vi "Config Main Error&Alarm.vi"(8 "error in (no error)":errorcluster, 11 "Sequence":T1) -> (0 "error out":errorcluster, 3 "Sequence out":T1)   [LabVIEW 2014, in "SeqLoop.lvlib"]
uses:
  TypeDefs/Sequence.ctl
  TypeDefs/STEP.ctl
  TypeDefs/LogicParsedExpression.ctl
  Mimico Display/TypeDefs/Mimic Data.ctl
  Mimico Display/TypeDefs/BG Image.ctl
  Mimico Display/TypeDefs/mObject.ctl
  <vilib>/regexp/Match Regular Expression.xnode
  SeqLoop.lvlib
  Mimico Display/Mimico Display.lvlib
panel:
  in  "Mensaje de Error":string
  in  "Alarm Msj 4":string
  in  "Alarm Msj 3":string
  in  "Alarm Msj 2":string
  in  "Alarm Msj 1":string
  in  "Alarm 4":string
  in  "Alarm 3":string
  in  "Alarm 2":string
  in  "Alarm 1":string
  in  "Condición de Error":string
  in  "Stop Med":bool
  in  "Add Med":bool
  # "Alarma"
  # "Mensaje de Alarma"
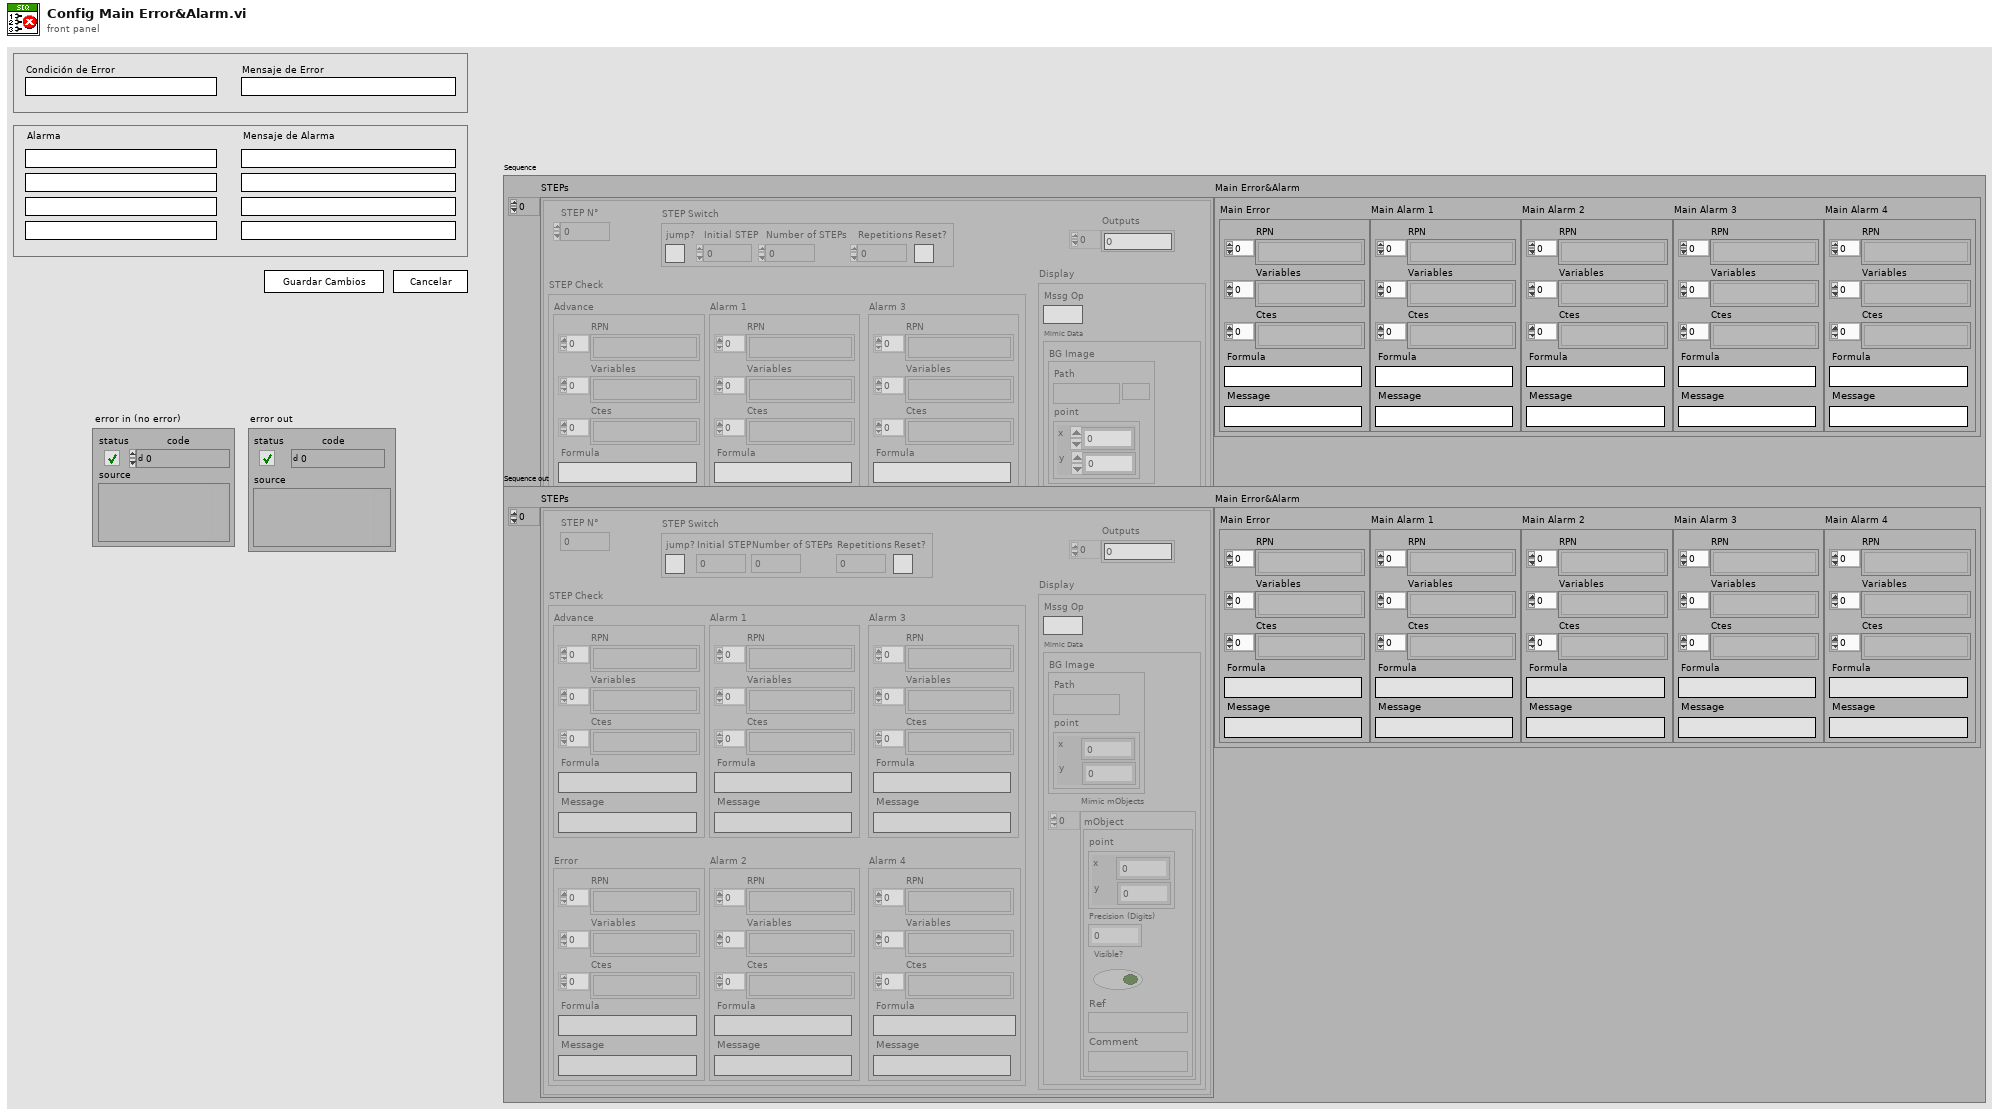
[diagram p1: front panel]
types:
  T1 = typedef "SeqLoop.lvlib/Sequence.ctl" = cluster{"STEPs":T2[], "Main Error&Alarm":cluster{"Main Error":T3, "Main Alarm 1":T3, "Main Alarm 2":T3, "Main Alarm 3":T3, "Main Alarm 4":T3}}
  T2 = typedef "SeqLoop.lvlib/STEP.ctl" = cluster{"STEP N°":u32, "STEP Switch":cluster{"jump?":bool, "Initial STEP":u32, "Number of STEPs":u32, "Repetitions":u32, "Reset?":bool}, "Outputs":i32[], "STEP Check":cluster{"Advance":T3, "Error ":T3, "Alarm 1":T3, "Alarm 2":T3, "Alarm 3":T3, "Alarm 4":T3}, "Display":cluster{"Mssg Op":string, "Mimic Data":T4}}
  T3 = typedef "SeqLoop.lvlib/LogicParsedExpression.ctl" = cluster{"RPN ":string[], "Variables":string[], "Ctes":string[], "Formula":string, "Message":string}
  T4 = typedef "SeqLoop.lvlib/Mimico Display.lvlib/Mimic Data.ctl" = cluster{"BG Image":T5, "Mimic mObjects":T6[]}
  T5 = typedef "SeqLoop.lvlib/Mimico Display.lvlib/BG Image.ctl" = cluster{"Path":path, "point":cluster{"x":i16, "y":i16}}
  T6 = typedef "SeqLoop.lvlib/Mimico Display.lvlib/mObject.ctl" = cluster{"point":cluster{"x":i16, "y":i16}, "Precision (Digits)":i32, "Visible?":bool, "Ref":string, "Comment":string}
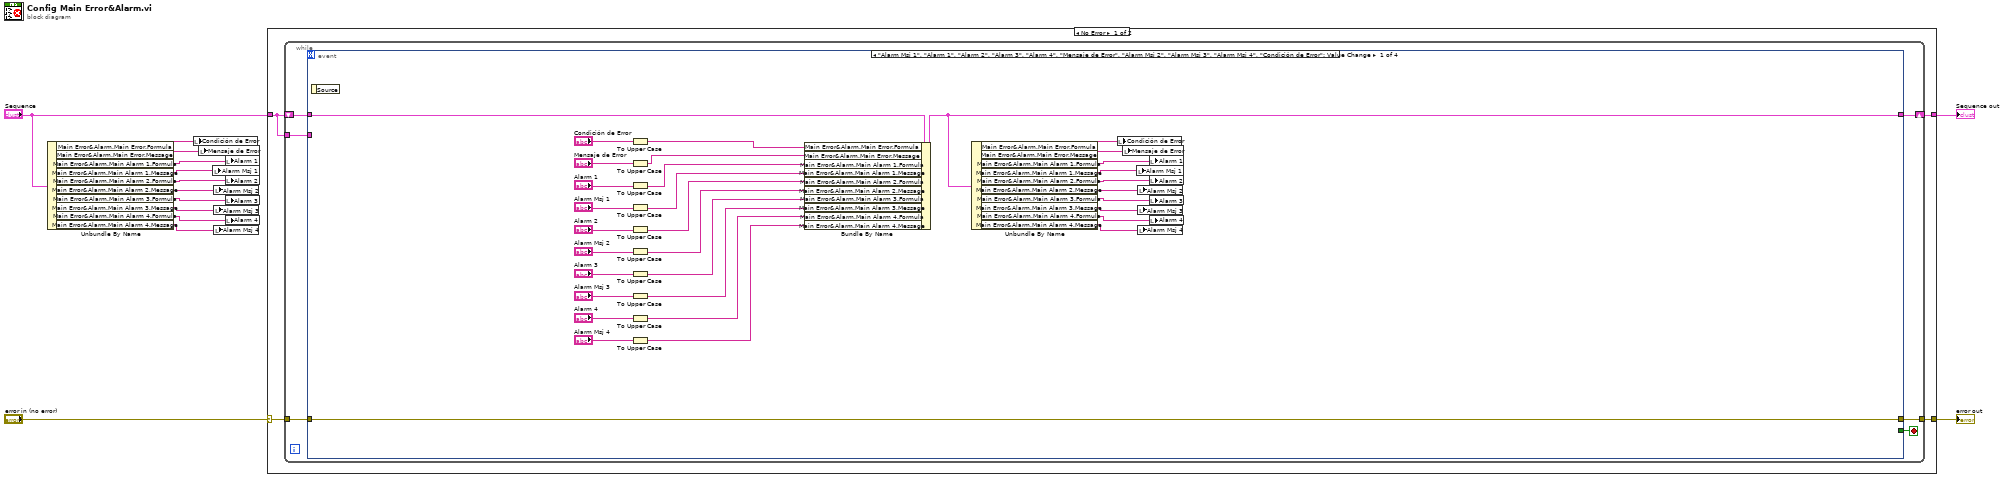
[diagram p0: block diagram]
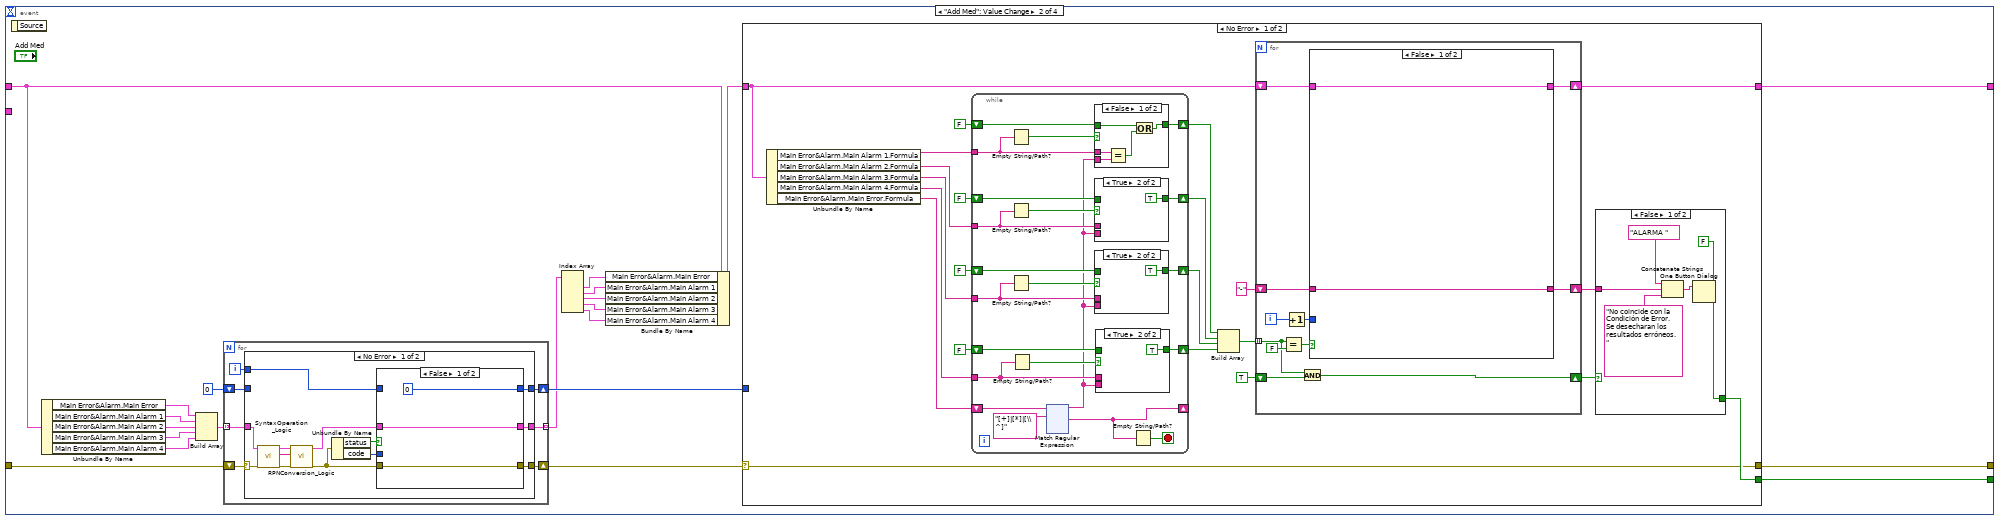
[diagram p2: hidden frame]
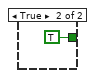
[diagram p3: hidden frame]
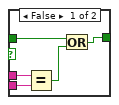
[diagram p4: hidden frame]
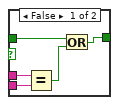
[diagram p5: hidden frame]
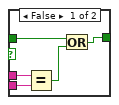
[diagram p6: hidden frame]
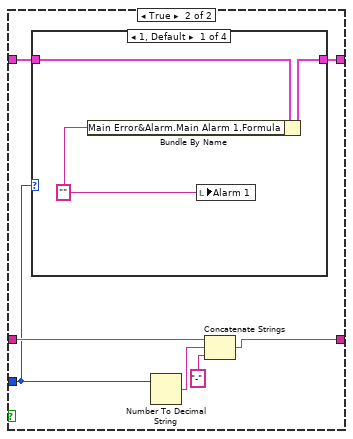
[diagram p7: hidden frame]
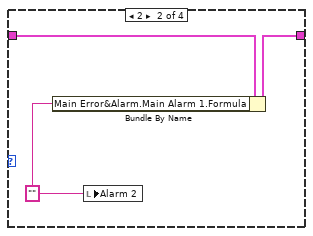
[diagram p8: hidden frame]
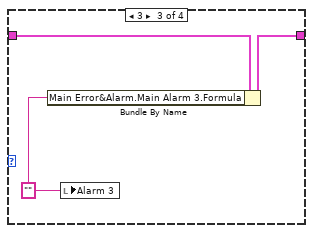
[diagram p9: hidden frame]
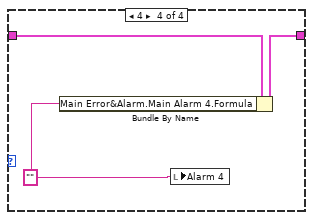
[diagram p10: hidden frame]
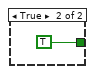
[diagram p11: hidden frame]
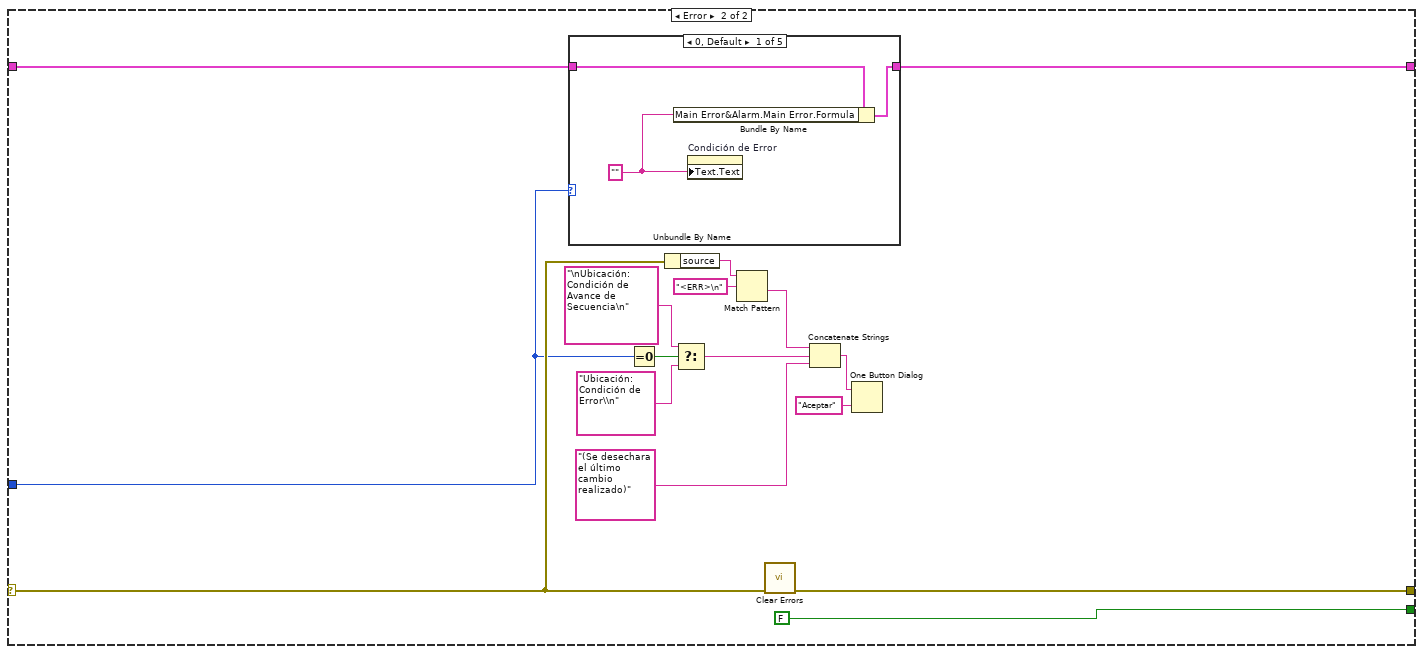
[diagram p12: hidden frame]
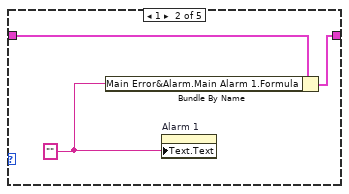
[diagram p13: hidden frame]
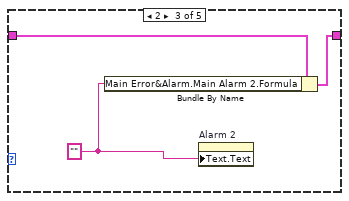
[diagram p14: hidden frame]
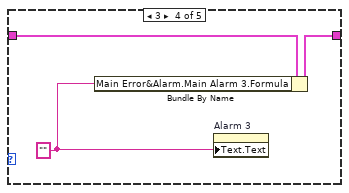
[diagram p15: hidden frame]
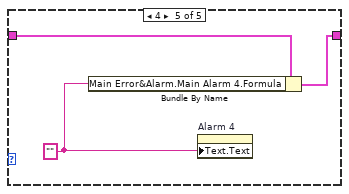
[diagram p16: hidden frame]
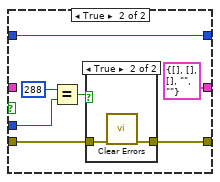
[diagram p17: hidden frame]
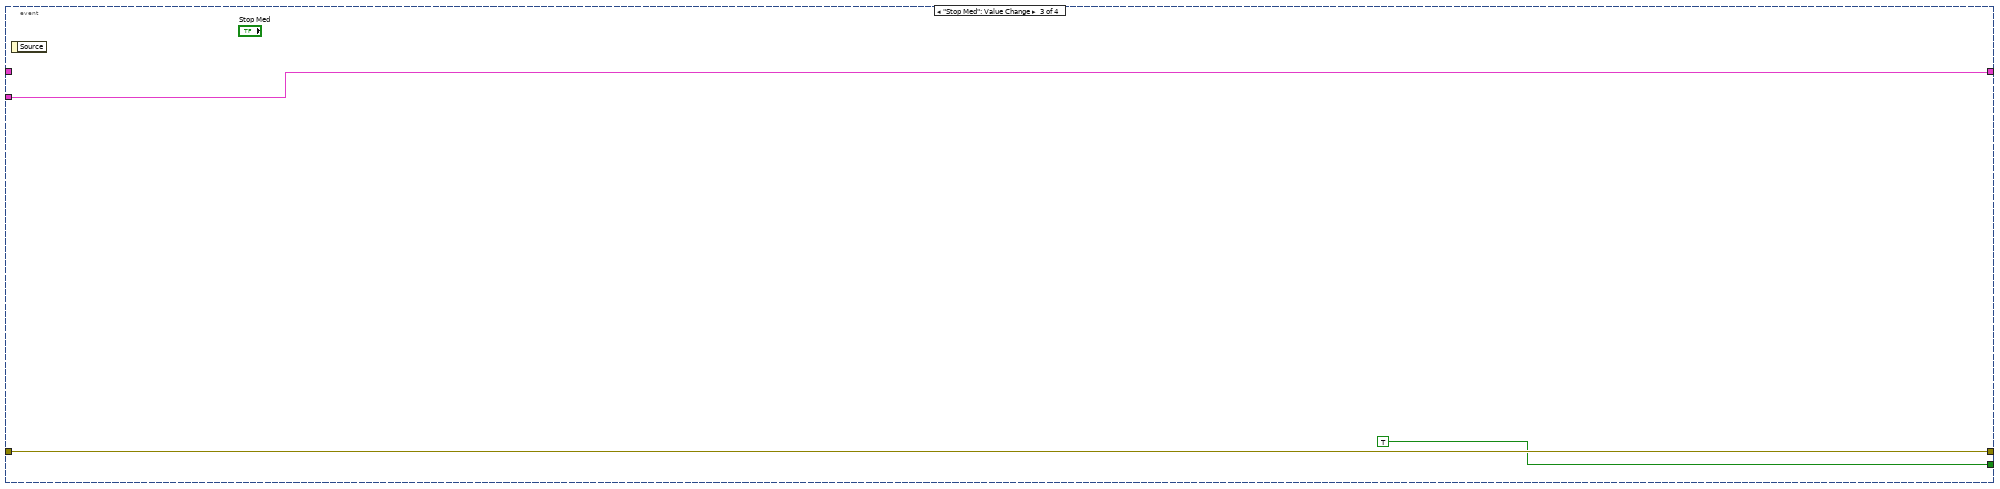
[diagram p20: hidden frame]
diagram:
  n1 = Unbundle By Name("Sequence") -> ("Main Error&Alarm.Main Error.Formula"=w11:string, "Main Error&Alarm.Main Error.Message"=w10:string, "Main Error&Alarm.Main Alarm 1.Formula"=w6:string, "Main Error&Alarm.Main Alarm 1.Message"=w5:string, "Main Error&Alarm.Main Alarm 2.Formula"=w4:string, "Main Error&Alarm.Main Alarm 2.Message"=w3:string, "Main Error&Alarm.Main Alarm 3.Formula"=w2:string, "Main Error&Alarm.Main Alarm 3.Message"=w7:string, "Main Error&Alarm.Main Alarm 4.Formula"=w8:string, "Main Error&Alarm.Main Alarm 4.Message"=w9:string)
  n2 = local write "Condición de Error"(w11) -> ()
  n3 = local write "Mensaje de Error"(w10) -> ()
  n4 = local write "Alarm Msj 1"(w5) -> ()
  n5 = local write "Alarm Msj 2"(w3) -> ()
  n6 = local write "Alarm Msj 3"(w7) -> ()
  n7 = local write "Alarm Msj 4"(w9) -> ()
  n8 = local write "Alarm 1"(w6) -> ()
  n9 = local write "Alarm 2"(w4) -> ()
  n10 = local write "Alarm 3"(w2) -> ()
  n11 = local write "Alarm 4"(w8) -> ()
  n12 = case shown="No Error" "error in (no error)" {
    selector: "error in (no error)" -> [w18 w373]
    tunnel: [w17 w373] -> w13
    tunnel: "Sequence" -> [w15 w372]
    tunnel: [w16 w372] -> w12
    frame No Error {
      n13 = while {
        tunnel: w18 -> [w24]
        tunnel: [w23] -> w17
        shift-right: [w19] -> w16
        shift-left: w15 -> [w21]
        tunnel: w15 -> [w20]
        stop <- w22 stop-if-true
        n14 = event shown="[0] \"Alarm Msj 1\", \"Alarm 1\", \"Alarm 2\", \"Alarm 3\", \"Alarm 4\", \"Mensaje de Error\", \"Alarm Msj 2\", \"Alarm Msj 3\", \"Alarm Msj 4\", \"Condición de Error\": Value Change" {
          selector: _ -> [_ _ _ _]
          dyn-events: _ -> [_ _ _ _]
          timeout: _ -> [_ _ _ _]
          tunnel: w24 -> [w57 w69 w366 w369]
          tunnel: [w57 w66 w366 w369] -> w23
          tunnel: [_ w68 TRUE ("Discard?") TRUE ("Discard?")] -> w22
          tunnel: w21 -> [w56 w65 _ _]
          tunnel: w20 -> [_ _ w367 w368]
          tunnel: [w45 w67 w367 w368] -> w19
          event "Alarm Msj 1", "Alarm 1", "Alarm 2", "Alarm 3", "Alarm 4", "Mensaje de Error", "Alarm Msj 2", "Alarm Msj 3", "Alarm Msj 4", "Condición de Error": Value Change {
            n15 = event-data() -> ()  [unwired: 1 in, 1 out]
            n16 = To Upper Case(1:"Condición de Error") -> (0:w25:string)
            n17 = To Upper Case(1:"Mensaje de Error") -> (0:w27:string)
            n18 = To Upper Case(1:"Alarm 1") -> (0:w29:string)
            n19 = To Upper Case(1:"Alarm Msj 1") -> (0:w31:string)
            n20 = To Upper Case(1:"Alarm 2") -> (0:w33:string)
            n21 = To Upper Case(1:"Alarm Msj 2") -> (0:w35:string)
            n22 = To Upper Case(1:"Alarm 3") -> (0:w37:string)
            n23 = To Upper Case(1:"Alarm Msj 3") -> (0:w39:string)
            n24 = To Upper Case(1:"Alarm 4") -> (0:w41:string)
            n25 = To Upper Case(1:"Alarm Msj 4") -> (0:w43:string)
            n26 = Bundle By Name(cluster=w56, "Main Error&Alarm.Main Error.Formula"=w25, "Main Error&Alarm.Main Error.Message"=w27, "Main Error&Alarm.Main Alarm 1.Formula"=w29, "Main Error&Alarm.Main Alarm 1.Message"=w31, "Main Error&Alarm.Main Alarm 2.Formula"=w33, "Main Error&Alarm.Main Alarm 2.Message"=w35, "Main Error&Alarm.Main Alarm 3.Formula"=w37, "Main Error&Alarm.Main Alarm 3.Message"=w39, "Main Error&Alarm.Main Alarm 4.Formula"=w41, "Main Error&Alarm.Main Alarm 4.Message"=w43) -> (w45:T1)
            n27 = Unbundle By Name(w45) -> ("Main Error&Alarm.Main Error.Formula"=w46:string, "Main Error&Alarm.Main Error.Message"=w47:string, "Main Error&Alarm.Main Alarm 1.Formula"=w51:string, "Main Error&Alarm.Main Alarm 1.Message"=w52:string, "Main Error&Alarm.Main Alarm 2.Formula"=w53:string, "Main Error&Alarm.Main Alarm 2.Message"=w54:string, "Main Error&Alarm.Main Alarm 3.Formula"=w55:string, "Main Error&Alarm.Main Alarm 3.Message"=w50:string, "Main Error&Alarm.Main Alarm 4.Formula"=w49:string, "Main Error&Alarm.Main Alarm 4.Message"=w48:string)
            n28 = local write "Condición de Error"(w46) -> ()
            n29 = local write "Mensaje de Error"(w47) -> ()
            n30 = local write "Alarm Msj 1"(w52) -> ()
            n31 = local write "Alarm Msj 2"(w54) -> ()
            n32 = local write "Alarm Msj 3"(w50) -> ()
            n33 = local write "Alarm Msj 4"(w48) -> ()
            n34 = local write "Alarm 1"(w51) -> ()
            n35 = local write "Alarm 2"(w53) -> ()
            n36 = local write "Alarm 3"(w55) -> ()
            n37 = local write "Alarm 4"(w49) -> ()
          }
          event "Add Med": Value Change {
            n38 = event-data() -> ()  [unwired: 1 in, 1 out]
            n39 = Unbundle By Name(w65) -> ("Main Error&Alarm.Main Error"=w78:T3, "Main Error&Alarm.Main Alarm 1"=w77:T3, "Main Error&Alarm.Main Alarm 2"=w76:T3, "Main Error&Alarm.Main Alarm 3"=w75:T3, "Main Error&Alarm.Main Alarm 4"=w74:T3)
            n40 = Build Array(w78, w77, w76, w75, w74) -> (w70:T3[])
            n41 = for {
              tunnel: w70 -> [w335] mode=indexing
              shift-right: [w334] -> w73
              shift-left: w69 -> [w332]
              shift-right: [w331] -> w72
              shift-left: 0 -> [w330]
              tunnel: [w329] -> w63 mode=indexing
              i -> [w333]
              n42 = case shown="No Error" w332 {
                selector: w332 -> [w345 w364]
                tunnel: w335 -> [w342 w362]
                tunnel: [w347 w364] -> w334
                tunnel: w333 -> [w346 _]
                tunnel: [w344 w363] -> w331
                tunnel: w330 -> [_ w363]
                tunnel: [w336 w362] -> w329
                frame No Error {
                  n43 = call "SyntaxOperation_Logic.vi"("error in (no error)"=w345, "Logical Parsed Expression"=w342) -> ("error out"=w341:errorcluster, "Token"=w339:string[], "Logical Parsed Expression Out"=w338:T3)  [unwired: 6 in, 1 out]
                  n44 = call "RPNConversion_Logic.vi"("error in"=w341, "Token"=w339, "Logical Parsed Expression"=w338) -> ("error out"=w340:errorcluster, "Logical Parsed Expression Out"=w337:T3)  [unwired: 7 in]
                  n45 = Unbundle By Name(w340) -> ("status"=w348:bool, "code"=w343:i32)
                  n46 = case shown="False" w348 {
                    tunnel: [w351 w353] -> w347
                    tunnel: w340 -> [w351 w354]
                    tunnel: w346 -> [_ w358]
                    tunnel: [0 w358] -> w344
                    tunnel: w343 -> [_ w357]
                    tunnel: w337 -> [w349 _]
                    tunnel: [w349 T3 {"RPN "=[], "Variables"=[], "Ctes"=[], "Formula"="", "Message"=""} ("Logical Parsed Expression Out")] -> w336
                    frame False {
                    }
                    frame True {
                      n47 = Equal?(x=288, y=w357) -> (x = y?=w355:bool)
                      n48 = case shown="True" w355 {
                        tunnel: w354 -> [w359 w361]
                        tunnel: [w359 w360] -> w353
                        frame False {
                        }
                        frame True {
                          n49 = call <vilib>:"Clear Errors.vi"("error in (no error)"=w361) -> ("error out"=w360:errorcluster)  [unwired: 5 in, 1 out]
                        }
                      }
                    }
                  }
                }
                frame Error {
                }
              }
            }
            n50 = Index Array(array=w63) -> (element #1=w62:T3, element #2=w59:T3, element #3=w58:T3, element #4=w60:T3, element #5=w61:T3)  [unwired: 5 in]
            n51 = Bundle By Name(cluster=w65, "Main Error&Alarm.Main Error"=w62, "Main Error&Alarm.Main Alarm 1"=w59, "Main Error&Alarm.Main Alarm 2"=w58, "Main Error&Alarm.Main Alarm 3"=w60, "Main Error&Alarm.Main Alarm 4"=w61) -> (w64:T1)
            n52 = case shown="No Error" w73 {
              selector: w73 -> [w85 w308]
              tunnel: [w96 w304] -> w67
              tunnel: w64 -> [w84 w305]
              tunnel: [w85 w307] -> w66
              tunnel: [w95 FALSE ("Discard?")] -> w68
              tunnel: w72 -> [_ w301]
              frame No Error {
                n53 = Unbundle By Name(w84) -> ("Main Error&Alarm.Main Alarm 1.Formula"=w83:string, "Main Error&Alarm.Main Alarm 2.Formula"=w82:string, "Main Error&Alarm.Main Alarm 3.Formula"=w81:string, "Main Error&Alarm.Main Alarm 4.Formula"=w80:string, "Main Error&Alarm.Main Error.Formula"=w79:string)
                n54 = while {
                  shift-right: [w101] -> _
                  shift-left: w79 -> [w103]
                  tunnel: w80 -> [w120]
                  tunnel: w81 -> [w113]
                  tunnel: w82 -> [w112]
                  tunnel: w83 -> [w111]
                  shift-right: [w119] -> w87
                  shift-left: FALSE -> [w118]
                  shift-right: [w108] -> w88
                  shift-left: FALSE -> [w105]
                  shift-right: [w109] -> w89
                  shift-left: FALSE -> [w106]
                  shift-right: [w110] -> w90
                  shift-left: FALSE -> [w107]
                  stop <- w117 stop-if-true
                  n55 = Empty String/Path?(string/path=w111) -> (empty?=w114:bool)
                  n56 = Empty String/Path?(string/path=w112) -> (empty?=w115:bool)
                  n57 = Empty String/Path?(string/path=w113) -> (empty?=w116:bool)
                  n58 = Empty String/Path?(string/path=w120) -> (empty?=w121:bool)
                  n59 = xnode "Match Regular Expression"("input string"=w103, "regular expression"="[+]|[*]|[\\^]") -> ("before match"=w102:string, "after match"=w101:string)  [unwired: 4 in, 3 out]
                  n60 = case shown="False" w114 {
                    tunnel: w111 -> [w240 _]
                    tunnel: w102 -> [w239 _]
                    tunnel: w107 -> [w238 _]
                    tunnel: [w236 TRUE] -> w110
                    frame False {
                      n61 = Equal?(x=w240, y=w239) -> (x = y?=w237:bool)
                      n62 = Or(x=w238, y=w237) -> (x .or. y?=w236:bool)
                    }
                    frame True {
                    }
                  }
                  n63 = case shown="True" w115 {
                    tunnel: w112 -> [w246 _]
                    tunnel: w102 -> [w245 _]
                    tunnel: w106 -> [w244 _]
                    tunnel: [w242 TRUE] -> w109
                    frame False {
                      n64 = Equal?(x=w246, y=w245) -> (x = y?=w243:bool)
                      n65 = Or(x=w244, y=w243) -> (x .or. y?=w242:bool)
                    }
                    frame True {
                    }
                  }
                  n66 = case shown="True" w116 {
                    tunnel: w113 -> [w252 _]
                    tunnel: w102 -> [w251 _]
                    tunnel: w105 -> [w250 _]
                    tunnel: [w248 TRUE] -> w108
                    frame False {
                      n67 = Equal?(x=w252, y=w251) -> (x = y?=w249:bool)
                      n68 = Or(x=w250, y=w249) -> (x .or. y?=w248:bool)
                    }
                    frame True {
                    }
                  }
                  n69 = case shown="True" w121 {
                    tunnel: w120 -> [w258 _]
                    tunnel: w102 -> [w257 _]
                    tunnel: w118 -> [w256 _]
                    tunnel: [w254 TRUE] -> w119
                    frame False {
                      n70 = Equal?(x=w258, y=w257) -> (x = y?=w255:bool)
                      n71 = Or(x=w256, y=w255) -> (x .or. y?=w254:bool)
                    }
                    frame True {
                    }
                  }
                  n72 = Empty String/Path?(string/path=w101) -> (empty?=w117:bool)
                }
                n73 = Build Array(w90, w89, w88, w87) -> (w86:bool[])
                n74 = for {
                  tunnel: w86 -> [w262] mode=indexing
                  shift-right: [w270] -> w99
                  shift-left: TRUE -> [w263]
                  shift-right: [w264] -> w97
                  shift-left: "-" ("string") -> [w265]
                  shift-right: [w261] -> w96
                  shift-left: w84 -> [w260]
                  i -> [w267]
                  n75 = Equal?(x=w262, y=FALSE) -> (x = y?=w268:bool)
                  n76 = Increment(x=w267) -> (x+1=w266:i32)
                  n77 = And(x=w262, y=w263) -> (x .and. y?=w270:bool)
                  n78 = case shown="False" w268 {
                    tunnel: w266 -> [_ w275]
                    tunnel: w265 -> [w272 w278]
                    tunnel: [w272 w277] -> w264
                    tunnel: [w271 w274] -> w261
                    tunnel: w260 -> [w271 w273]
                    frame False {
                    }
                    frame True {
                      n79 = case shown="1, Default" w275 {
                        tunnel: [w282 w285 w288 w291] -> w274
                        tunnel: w273 -> [w281 w284 w287 w290]
                        frame 1, Default {
                          w280 = "" ("Alarm 1.Formula")
                          n80 = Bundle By Name(cluster=w281, "Main Error&Alarm.Main Alarm 1.Formula"=w280) -> (w282:T1)
                          n81 = local write "Alarm 1"(w280) -> ()
                        }
                        frame 2 {
                          w283 = "" ("Alarm 1.Formula")
                          n82 = Bundle By Name(cluster=w284, "Main Error&Alarm.Main Alarm 1.Formula"=w283) -> (w285:T1)
                          n83 = local write "Alarm 2"(w283) -> ()
                        }
                        frame 3 {
                          w286 = "" ("Alarm 1.Formula")
                          n84 = Bundle By Name(cluster=w287, "Main Error&Alarm.Main Alarm 3.Formula"=w286) -> (w288:T1)
                          n85 = local write "Alarm 3"(w286) -> ()
                        }
                        frame 4 {
                          w289 = "" ("Alarm 1.Formula")
                          n86 = Bundle By Name(cluster=w290, "Main Error&Alarm.Main Alarm 4.Formula"=w289) -> (w291:T1)
                          n87 = local write "Alarm 4"(w289) -> ()
                        }
                      }
                      n88 = Number To Decimal String(number=w275) -> (decimal integer string=w279:string)  [unwired: 1 in]
                      n89 = Concatenate Strings(w278, w279, "-" ("string")) -> (w277:string)
                    }
                  }
                }
                n90 = case shown="False" w99 {
                  tunnel: [FALSE TRUE] -> w95
                  tunnel: w97 -> [w294 _]
                  frame False {
                    n91 = Concatenate Strings("ALARMA " ("message"), w294, "No coincide con la Condición de Error. Se desecharan los resultados erróneos." ("string")) -> (w293:string)
                    n92 = One Button Dialog(message=w293) -> ()  [unwired: 1 in, 1 out]
                  }
                  frame True {
                  }
                }
              }
              frame Error {
                n93 = case shown="0, Default" w301 {
                  tunnel: w305 -> [w316 w319 w322 w325 w328]
                  tunnel: [w315 w318 w321 w324 w327] -> w304
                  frame 0, Default {
                    w314 = "" ("Text.Text")
                    n94 = Bundle By Name(cluster=w316, "Main Error&Alarm.Main Error.Formula"=w314) -> (w315:T1)
                    n95 = property on="Condición de Error" class="Str"("Text.Text"=w314) -> ()  [unwired: 2 in, 2 out]
                  }
                  frame 1 {
                    w317 = "" ("Text.Text")
                    n96 = Bundle By Name(cluster=w319, "Main Error&Alarm.Main Alarm 1.Formula"=w317) -> (w318:T1)
                    n97 = property on="Alarm 1" class="Str"("Text.Text"=w317) -> ()  [unwired: 2 in, 2 out]
                  }
                  frame 2 {
                    w320 = "" ("Text.Text")
                    n98 = Bundle By Name(cluster=w322, "Main Error&Alarm.Main Alarm 2.Formula"=w320) -> (w321:T1)
                    n99 = property on="Alarm 2" class="Str"("Text.Text"=w320) -> ()  [unwired: 2 in, 2 out]
                  }
                  frame 3 {
                    w323 = "" ("Text.Text")
                    n100 = Bundle By Name(cluster=w325, "Main Error&Alarm.Main Alarm 3.Formula"=w323) -> (w324:T1)
                    n101 = property on="Alarm 3" class="Str"("Text.Text"=w323) -> ()  [unwired: 2 in, 2 out]
                  }
                  frame 4 {
                    w326 = "" ("Text.Text")
                    n102 = Bundle By Name(cluster=w328, "Main Error&Alarm.Main Alarm 4.Formula"=w326) -> (w327:T1)
                    n103 = property on="Alarm 4" class="Str"("Text.Text"=w326) -> ()  [unwired: 2 in, 2 out]
                  }
                }
                n104 = Equal To 0?(x=w301) -> (x = 0?=w302:bool)
                n105 = Unbundle By Name(w308) -> ("source"=w310:string)
                n106 = Select(t="\nUbicación: Condición de Avance de Secuencia\n" ("regular expression"), s=w302, f="Ubicación: Condición de Error\\n" ("regular expression")) -> (s? t:f=w300:string)
                n107 = Match Pattern(string=w310, regular expression="<ERR>\n") -> (after substring=w312:string)  [unwired: 1 in, 3 out]
                n108 = call <vilib>:"Clear Errors.vi"("error in (no error)"=w308) -> ("error out"=w307:errorcluster)  [unwired: 5 in, 1 out]
                n109 = Concatenate Strings(w312, w300, "(Se desechara el último cambio realizado)" ("button name (\"OK\")")) -> (w313:string)
                n110 = One Button Dialog(message=w313, button name ("OK")="Aceptar") -> ()  [unwired: 1 out]
              }
            }
          }
          event "Stop Med": Value Change {
            n111 = event-data() -> ()  [unwired: 1 in, 1 out]
          }
          event Panel Close? {
            n112 = event-data() -> ()  [unwired: 1 in, 1 out]
            n113 = event-data("Discard?"=TRUE) -> ()  [unwired: 1 in, 1 out]
          }
        }
      }
    }
    frame Error {
    }
  }
  "error out" <- w13
  "Sequence out" <- w12
